vi "DSF.Shared.Configuration.Transfer Group.Create.vi"(8 "error in (no error)":errorcluster, 11 "Transfer Group Configuration cluster":T1={"name"="", "direction"=enum."Tx", "cycle timing"={"Priority"=0, "Decimation"=1, "Offset"=0}, "Transfers"=[]}) -> (0 "error out":errorcluster, 3 "Transfer Group Configuration":refnum<class "DSF.Shared.Configuration.Transfer Group.lvclass">)   [LabVIEW 2017, in "DSF.Engine.lvlib" / "DSF.Shared.Configuration.Transfer Group.lvclass"]
uses:
  DSF.Shared.Configuration.Transfer Group.lvclass
  Typedefs/DSF.Shared.Refactor.Typedefs.Transfer Group Configuration.Aggregate.ctl
  Typedefs/DSF.Shared.Typedefs.Direction.ctl
  Typedefs/DSF.Shared.Typedefs.Cycle Timing Factors.ctl
  Typedefs/DSF.Shared.Refactor.Typedefs.Transfer Configuration.ctl
  Typedefs/DSF.Shared.Typedefs.Byte Order.ctl
  Typedefs/DSF.Shared.Refactor.Typedefs.Channel Array Configuration.ctl
  Typedefs/DSF.Shared.Typedefs.Data Type.ctl
  DSF.Shared.Configuration.Transfer Group.lvclass/DSF.Shared.Configuration.Transfer Group.ctl
  Transfer/DSF.Shared.Configuration.Transfer.lvclass
  DSF.Engine.lvlib
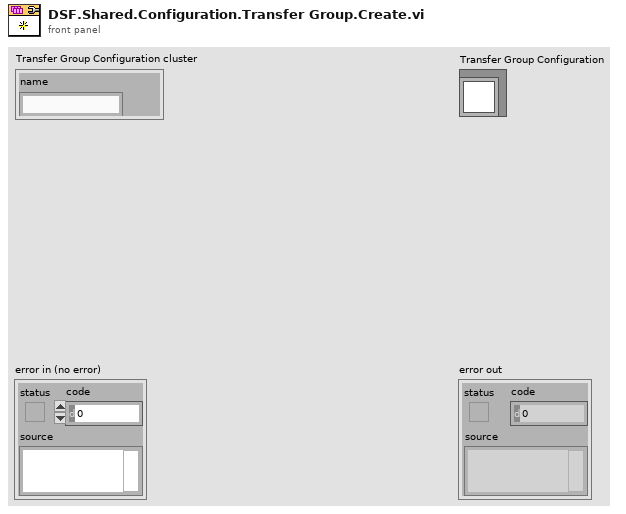
[diagram p1: front panel]
types:
  T1 = typedef "DSF.Engine.lvlib/DSF.Shared.Refactor.Typedefs.Transfer Group Configuration.Aggregate.ctl" = cluster{"name":string, "direction":T2, "cycle timing":T3, "Transfers":T4[]}
  T2 = typedef "DSF.Engine.lvlib/DSF.Shared.Typedefs.Direction.ctl" = enum8{"Tx", "Rx"}
  T3 = typedef "DSF.Engine.lvlib/DSF.Shared.Typedefs.Cycle Timing Factors.ctl" = cluster{"Priority":u64, "Decimation":u64, "Offset":u64}
  T4 = typedef "DSF.Engine.lvlib/DSF.Shared.Refactor.Typedefs.Transfer Configuration.ctl" = cluster{"name":string, "byte order":T5, "channel configurations":T6[]}
  T5 = typedef "DSF.Engine.lvlib/DSF.Shared.Typedefs.Byte Order.ctl" = enum8{"big-endian", "little-endian"}
  T6 = typedef "DSF.Engine.lvlib/DSF.Shared.Refactor.Typedefs.Channel Array Configuration.ctl" = cluster{"name":string, "data type":T7, "count":u64, "buffer offset":u64, "engine offset":u64}
  T7 = typedef "DSF.Engine.lvlib/DSF.Shared.Typedefs.Data Type.ctl" = enum8{"Bool", "SGL", "DBL", "I8", "I16", "I32", "I64", "U8", "U16", "U32", "U64"}
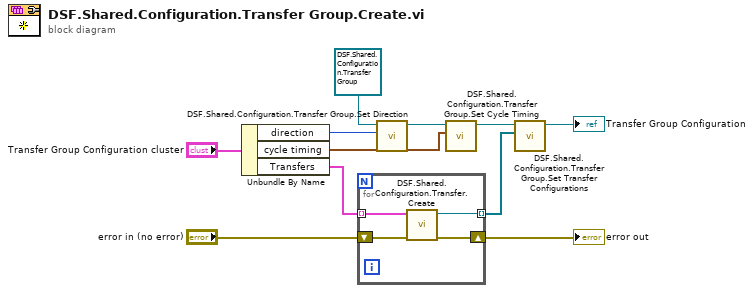
[diagram p0: block diagram]
diagram:
  n1 = Unbundle By Name("Transfer Group Configuration cluster") -> ("direction"=w5:T2, "cycle timing"=w4:T3, "Transfers"=w9:T4[])
  n2 = for {
    shift-right: [w13] -> w8
    shift-left: "error in (no error)" -> [w15]
    tunnel: w9 -> [w14] mode=indexing
    tunnel: [w12] -> w7 mode=indexing
    n3 = call "DSF.Shared.Configuration.Transfer.Create.vi"("error in (no error)"=w15, "Transfer Configuration cluster"=w14) -> ("error out"=w13:errorcluster, "Transfer Configuration out"=w12:refnum<class "DSF.Shared.Configuration.Transfer.lvclass">)  [unwired: 8 in]
  }
  "error out" <- w8
  n4 = call "DSF.Shared.Configuration.Transfer Group.Set Direction.vi"("direction"=w5, "Transfer Group Configuration in"=refnum<class "DSF.Shared.Configuration.Transfer Group.lvclass"> refnum) -> ("Transfer Group Configuration out"=w3:refnum<class "DSF.Shared.Configuration.Transfer Group.lvclass">)  [unwired: 9 in]
  n5 = call "DSF.Shared.Configuration.Transfer Group.Set Cycle Timing.vi"("cycle timing"=w4, "Transfer Group Configuration in"=w3) -> ("Transfer Group Configuration out"=w2:refnum<class "DSF.Shared.Configuration.Transfer Group.lvclass">)  [unwired: 9 in]
  n6 = call "DSF.Shared.Configuration.Transfer Group.Set Transfer Configurations.vi"("Transfer Configurations"=w7, "Transfer Group Configuration in"=w2) -> ("Transfer Group Configuration out"=→"Transfer Group Configuration":refnum<class "DSF.Shared.Configuration.Transfer Group.lvclass">)  [unwired: 9 in]
